vi "Calculate N_total and Updates.vi"(11 "Generator in":refnum<class "Generator.lvclass">) -> (1 "Updates":i32, 2 "Total Samples":i32, 3 "Samples/Update":i32)   [LabVIEW 2019, in "Generator.lvclass"]
uses:
  Generator.lvclass
  Generator.lvclass/Generator.ctl
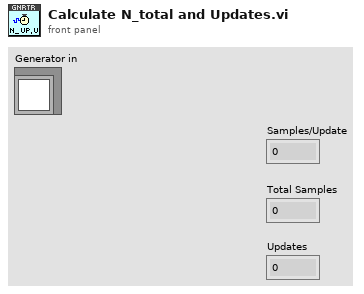
[diagram p1: front panel]
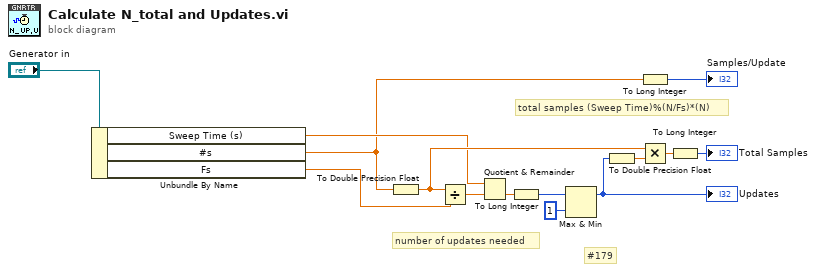
[diagram p0: block diagram]
diagram:
  # "#179"
  # "number of updates needed"
  # "total samples (Sweep Time)%(N/Fs)*(N)"
  n1 = Unbundle By Name("Generator in") -> ("Sweep Time (s)"=w6:dbl, "#s"=w5:dbl, "Fs"=w7:dbl)
  n2 = To Double Precision Float(number=w5) -> (double precision float=w11:dbl)
  n3 = Divide(x=w11, y=w7) -> (x/y=w12:dbl)
  n4 = Quotient & Remainder(x=w6, y=w12) -> (floor(x/y)=w13:dbl)  [unwired: 1 out]
  n5 = To Long Integer(number=w13) -> (32bit integer=w3:i32)
  n6 = Max & Min(x=w3, y=1) -> (max(x,y)=w1:i32)  [unwired: 1 out]
  "Updates" <- w1
  n7 = To Double Precision Float(number=w1) -> (double precision float=w9:dbl)
  n8 = To Long Integer(number=w5) -> (32bit integer=→"Samples/Update":i32)
  n9 = Multiply(x=w11, y=w9) -> (x*y=w14:dbl)
  n10 = To Long Integer(number=w14) -> (32bit integer=→"Total Samples":i32)
